vi "Get Double Array.vi"(8 "error in (no error)":errorcluster, 11 "Array in":refnum<class "Array.lvclass">) -> (0 "error out":errorcluster, 1 "Array dimensions":i32[](array[numeric]), 2 "DBL array out":dbl[](array[numeric]), 3 "Array out":refnum<class "Array.lvclass">)   [LabVIEW 2013, in "MDSplus.lvlib" / "Array.lvclass"]
uses:
  <vilib>/MDSplus/Classes/Data_Class/Array_Class/Array.lvclass
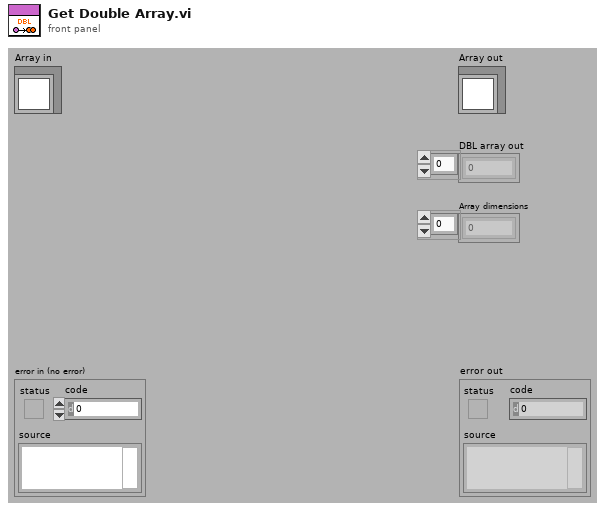
[diagram p1: front panel]
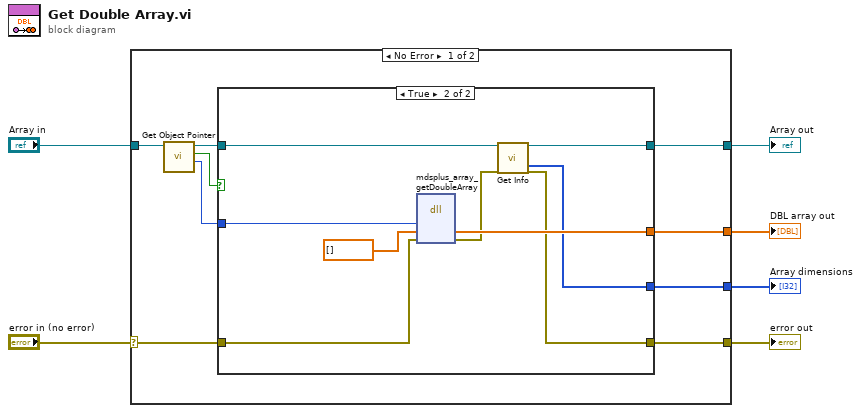
[diagram p0: block diagram]
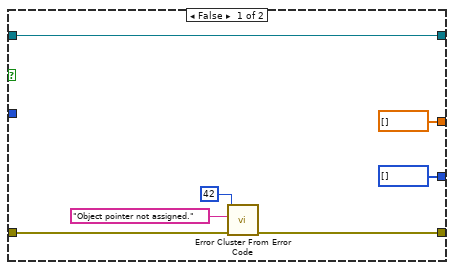
[diagram p2: hidden frame]
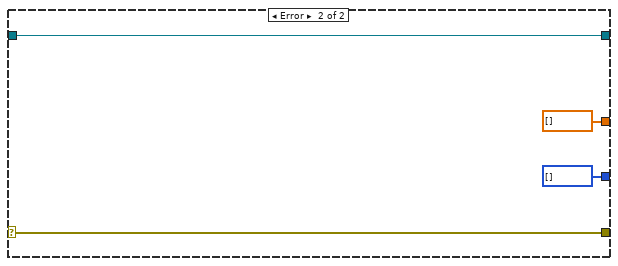
[diagram p3: hidden frame]
diagram:
  n1 = case shown="No Error" "error in (no error)" {
    selector: "error in (no error)" -> [w10 w35]
    tunnel: [w9 w35] -> w5
    tunnel: [w8 w34] -> w3
    tunnel: "Array in" -> [w15 w34]
    tunnel: [w14 dbl[] [] ("lvFltArrHdlOut")] -> w2
    tunnel: [w7 i32[] [] ("Dimensions out")] -> w1
    frame No Error {
      n2 = call-dynamic "Get Object Pointer.vi"("Data in"=w15) -> ("Object Pointer"=w12:i64, "Assigned object pointer?"=w13:bool, "Data out"=w11:refnum<class "Array.lvclass">)  [unwired: 8 in]
      n3 = case shown="True" w13 {
        tunnel: [dbl[] [] ("lvFltArrHdlOut") w30] -> w14
        tunnel: w12 -> [_ w29]
        tunnel: w11 -> [w22 w27]
        tunnel: w10 -> [w17 w28]
        tunnel: [w16 w24] -> w9
        tunnel: [w22 w26] -> w8
        tunnel: [i32[] [] ("Dimensions out") w23] -> w7
        frame False {
          n4 = call <vilib>:"Error Cluster From Error Code.vi"("error in (no error)"=w17, "error message (\"\")"="Object pointer not assigned." ("error message (\"\")"), "error code (0)"=42) -> ("error out"=w16:errorcluster)  [unwired: 6 in]
        }
        frame True {
          n5 = dll-call lib="MDSobjectsLVShr" fn="mdsplus_array_getDoubleArray"("lvArrayPtr"=w29, "lvDblArrHdlOut"=dbl[] [] ("floatOut"), "error"=w28) -> ("lvDblArrHdlOut"=w30:dbl[], "error"=w25:errorcluster)  [unwired: 5 in, 2 out]
          n6 = call-dynamic "Get Info.vi"("Array in"=w27, "error in (no error)"=w25) -> ("Array out"=w26:refnum<class "Array.lvclass">, "Dimensions out"=w23:i32[], "error out"=w24:errorcluster)  [unwired: 12 in, 3 out]
        }
      }
    }
    frame Error {
    }
  }
  "error out" <- w5
  "Array out" <- w3
  "DBL array out" <- w2
  "Array dimensions" <- w1
